vi "set RP100 voltage.vi"(8 "error in (no error)":errorcluster, 10 "字符串 2":string, 11 "config":T1={"initialize"=enum."SR830", "6221"={"6221 Resource"="GPIB0::24::INSTR", "Delta status"=FALSE, "电流|RMS(A)"=0.0}, "SR830+6221"={"source"=0, "Current(A)"=0.0, "阻抗(Ohm)"=0.0, "SR830 1"=FALSE, "SR830 2"=FALSE, "SR830 3"=FALSE, "SR830 4"=FALSE, "VISA 1"="", "VISA 2"="", "VISA 3"="", "VISA 4"="", "Reserve 1"=-1, "Reserve 2"=-1, "Reserve 3"=-1, "Reserve 4"=-1, "Sensitivity 1"=-1, "Sensitivity 2"=-1, "Sensitivity 3"=-1, "Sensitivity 4"=-1, "量程入 1"=0, "量程入 2"=0, "量程入 3"=0, "量程入 4"=0}, "2400"={"2400"=FALSE, "VISA"="GPIB0::9::INSTR", "Output Level (0)"=1e-05, "Compliance  Level (0.1)"=10.0, "ch"=[]}, "ch"={"ch"=[], "current"=[], "change?"=[], "holding current\nwhen change ch?"=FALSE, "current offset"=[]}, "Instrument"={"limit"={"Field limit"=0.0, "Field rate limit"=0.0, "Temp limit"=0.0, "Temp low limit"=0.0, "Temp rate limit "=0.0}, "genarl"={"行数"=refnum, "编辑列表框？"=refnum, "列表框"=refnum, "camg 振荡状态"=refnum, "Aborting"=refnum, "数据文件"=refnum, "warning"=refnum, "vi路径"="", "Instrument Type"=enum."PPMS-Rotate"}, "cmag"={"TM620"="TCPIP0::192.168.1.5::4266::SOCKET", "M24C Resource"="GPIB0::24::INSTR", "4G supply"="", "Temp Status 24C"=refnum, "Temp"=refnum, "9T信号"=refnum, "4g supply status"=refnum, "in-plane"="", "out-plane"="", "in-plane signal"=FALSE, "out-plane signal"=FALSE, "in plane 信号"=refnum, "pzt volt"=refnum, "camg Rate"=refnum}, "lengtou2"={"750 visa"="", "750 rotate"="", "semaphore 340"=refnum, "semaphore 750"=refnum, "750 field status"=refnum, "Input (0:A) 340"=0, "340 Resource"="GPIB0::14::INSTR", "340 Status"=refnum, "Input (0:B) 340"=1, "Loop (0: 1)"=0, "Loop (1: 1)"=0, "TCP master instance"=refnum}, "lengtou"={"TCP master instance"=refnum, "335 Status"=refnum, "335 Resource "="GPIB0::24::INSTR", "Input (0:A) 335"=0, "Input (0:B) 335"=1, "Heater Output (1:1) 335"=1, "semaphore 335"=refnum}, "325 for test"={"quantum design"=refnum, "semaphore 325"=refnum, "325 Resource "="GPIB0::13::INSTR", "Input (0:A) 325"=0, "Heater Output (1:1) 325"=1, "325 Status"=refnum}}, "2614B"={"2614B chA"=FALSE, "2614B chB"=FALSE, "VISA"=""}, "33522b"={"33522b resource name"="GPIB0::16::INSTR", "零电压"=0.0, "最大电压"=148.0, "间隔"=4.0, "最小电压"=-48.0, "loop"=0.0, "压电陶瓷电压(Vpp)"=0.0}, "gating type"=enum."2614(daul)", "层数"=0, "行数"=0, "是否处理"=[], "current 2"=[], "StrainCell"={"RP100 resource name"="GPIB0::16::INSTR", "E4980 resource name"="GPIB0::16::INSTR", "RP100 Reset ?(True)"=TRUE, "Voltage1(V)"=0.0, "Voltage2(V)"=148.0, "interval"=4.0, "slew(V/s)"=-48.0}} {"Instrument"."325 for test"."Heater Output (1:1) 325" items=["1"=1, "2"=2]; "Instrument"."325 for test"."Input (0:A) 325" items=["A", "B"]; "Instrument"."lengtou"."Heater Output (1:1) 335" items=["1"=1, "2"=2]; "Instrument"."lengtou"."Input (0:B) 335" items=["A", "B"]; "Instrument"."lengtou"."Input (0:A) 335" items=["A", "B"]; "Instrument"."lengtou2"."Loop (1: 1)" items=["1", "2"]; "Instrument"."lengtou2"."Loop (0: 1)" items=["1", "2"]; "Instrument"."lengtou2"."Input (0:B) 340" items=["A", "B", "C", "D"]; "Instrument"."lengtou2"."Input (0:A) 340" items=["A", "B", "C", "D"]; "SR830+6221"."Sensitivity 4" items=["Auto Gain"=-1, "2 nV/fA"=0, "5 nV/fA"=1, "10 nV/fA"=2, "20 nV/fA"=3, "50 nV/fA"=4, "100 nV/fA"=5, "200 nV/fA"=6, "500 nV/fA"=7, "1 uV/pA"=8, "2 uV/pA"=9, "5 uV/pA"=10, "10 uV/pA"=11, "20 uV/pA"=12, "50 uV/pA"=13, "100 uV/pA"=14, "200 uV/pA"=15, "500 uV/pA"=16, "1 mV/nA"=17, "2 mV/nA"=18, "5 mV/nA"=19, "10 mV/nA"=20, "20 mV/nA"=21, "50 mV/nA"=22, "100 mV/nA"=23, "200 mV/nA"=24, "500 mV/mA"=25, "1 V/uA"=26]; "SR830+6221"."Sensitivity 3" items=["Auto Gain"=-1, "2 nV/fA"=0, "5 nV/fA"=1, "10 nV/fA"=2, "20 nV/fA"=3, "50 nV/fA"=4, "100 nV/fA"=5, "200 nV/fA"=6, "500 nV/fA"=7, "1 uV/pA"=8, "2 uV/pA"=9, "5 uV/pA"=10, "10 uV/pA"=11, "20 uV/pA"=12, "50 uV/pA"=13, "100 uV/pA"=14, "200 uV/pA"=15, "500 uV/pA"=16, "1 mV/nA"=17, "2 mV/nA"=18, "5 mV/nA"=19, "10 mV/nA"=20, "20 mV/nA"=21, "50 mV/nA"=22, "100 mV/nA"=23, "200 mV/nA"=24, "500 mV/mA"=25, "1 V/uA"=26]; "SR830+6221"."Sensitivity 1" items=["Auto Gain"=-1, "2 nV/fA"=0, "5 nV/fA"=1, "10 nV/fA"=2, "20 nV/fA"=3, "50 nV/fA"=4, "100 nV/fA"=5, "200 nV/fA"=6, "500 nV/fA"=7, "1 uV/pA"=8, "2 uV/pA"=9, "5 uV/pA"=10, "10 uV/pA"=11, "20 uV/pA"=12, "50 uV/pA"=13, "100 uV/pA"=14, "200 uV/pA"=15, "500 uV/pA"=16, "1 mV/nA"=17, "2 mV/nA"=18, "5 mV/nA"=19, "10 mV/nA"=20, "20 mV/nA"=21, "50 mV/nA"=22, "100 mV/nA"=23, "200 mV/nA"=24, "500 mV/mA"=25, "1 V/uA"=26]; "SR830+6221"."Sensitivity 2" items=["Auto Gain"=-1, "2 nV/fA"=0, "5 nV/fA"=1, "10 nV/fA"=2, "20 nV/fA"=3, "50 nV/fA"=4, "100 nV/fA"=5, "200 nV/fA"=6, "500 nV/fA"=7, "1 uV/pA"=8, "2 uV/pA"=9, "5 uV/pA"=10, "10 uV/pA"=11, "20 uV/pA"=12, "50 uV/pA"=13, "100 uV/pA"=14, "200 uV/pA"=15, "500 uV/pA"=16, "1 mV/nA"=17, "2 mV/nA"=18, "5 mV/nA"=19, "10 mV/nA"=20, "20 mV/nA"=21, "50 mV/nA"=22, "100 mV/nA"=23, "200 mV/nA"=24, "500 mV/mA"=25, "1 V/uA"=26]; "SR830+6221"."Reserve 4" items=["Auto Reserve"=-1, "High Reserve"=0, "Normal"=1, "Low Noise"=2]; "SR830+6221"."Reserve 3" items=["Auto Reserve"=-1, "High Reserve"=0, "Normal"=1, "Low Noise"=2]; "SR830+6221"."Reserve 2" items=["Auto Reserve"=-1, "High Reserve"=0, "Normal"=1, "Low Noise"=2]; "SR830+6221"."Reserve 1" items=["Auto Reserve"=-1, "High Reserve"=0, "Normal"=1, "Low Noise"=2]; "SR830+6221"."source" items=["SR830 1", "SR830 2", "SR830 3", "SR830 4"]}) -> (0 "error out":errorcluster, 3 "输出簇":T1={"initialize"=enum."SR830", "6221"={"6221 Resource"="GPIB0::24::INSTR", "Delta status"=FALSE, "电流|RMS(A)"=0.0}, "SR830+6221"={"source"=0, "Current(A)"=0.0, "阻抗(Ohm)"=0.0, "SR830 1"=FALSE, "SR830 2"=FALSE, "SR830 3"=FALSE, "SR830 4"=FALSE, "VISA 1"="", "VISA 2"="", "VISA 3"="", "VISA 4"="", "Reserve 1"=-1, "Reserve 2"=-1, "Reserve 3"=-1, "Reserve 4"=-1, "Sensitivity 1"=-1, "Sensitivity 2"=-1, "Sensitivity 3"=-1, "Sensitivity 4"=-1, "量程入 1"=0, "量程入 2"=0, "量程入 3"=0, "量程入 4"=0}, "2400"={"2400"=FALSE, "VISA"="GPIB0::9::INSTR", "Output Level (0)"=1e-05, "Compliance  Level (0.1)"=10.0, "ch"=[]}, "ch"={"ch"=[], "current"=[], "change?"=[], "holding current\nwhen change ch?"=FALSE, "current offset"=[]}, "Instrument"={"limit"={"Field limit"=0.0, "Field rate limit"=0.0, "Temp limit"=0.0, "Temp low limit"=0.0, "Temp rate limit "=0.0}, "genarl"={"行数"=refnum, "编辑列表框？"=refnum, "列表框"=refnum, "camg 振荡状态"=refnum, "Aborting"=refnum, "数据文件"=refnum, "warning"=refnum, "vi路径"="", "Instrument Type"=enum."PPMS-Rotate"}, "cmag"={"TM620"="GPIB0::24::INSTR", "M24C Resource"="GPIB0::24::INSTR", "4G supply"="GPIB0::24::INSTR", "Temp Status 24C"=refnum, "Temp"=refnum, "9T信号"=refnum, "4g supply status"=refnum, "in-plane"="", "out-plane"="", "in-plane signal"=FALSE, "out-plane signal"=FALSE, "in plane 信号"=refnum, "pzt volt"=refnum, "camg Rate"=refnum}, "lengtou2"={"750 visa"="", "750 rotate"="", "semaphore 340"=refnum, "semaphore 750"=refnum, "750 field status"=refnum, "Input (0:A) 340"=1, "340 Resource"="GPIB0::14::INSTR", "340 Status"=refnum, "Input (0:B) 340"=0, "Loop (0: 1)"=1, "Loop (1: 1)"=0, "TCP master instance"=refnum}, "lengtou"={"TCP master instance"=refnum, "335 Status"=refnum, "335 Resource "="GPIB0::24::INSTR", "Input (0:A) 335"=0, "Input (0:B) 335"=0, "Heater Output (1:1) 335"=0, "semaphore 335"=refnum}, "325 for test"={"quantum design"=refnum, "semaphore 325"=refnum, "325 Resource "="GPIB0::13::INSTR", "Input (0:A) 325"=1000, "Heater Output (1:1) 325"=1, "325 Status"=refnum}}, "2614B"={"2614B chA"=FALSE, "2614B chB"=FALSE, "VISA"=""}, "33522b"={"33522b resource name"="GPIB0::16::INSTR", "零电压"=0.0, "最大电压"=148.0, "间隔"=4.0, "最小电压"=-48.0, "loop"=0.0, "压电陶瓷电压(Vpp)"=0.0}, "gating type"=enum."2614(daul)", "层数"=0, "行数"=0, "是否处理"=[], "current 2"=[], "StrainCell"={"RP100 resource name"="GPIB0::16::INSTR", "E4980 resource name"="GPIB0::16::INSTR", "RP100 Reset ?(True)"=TRUE, "Voltage1(V)"=0.0, "Voltage2(V)"=0.0, "interval"=4.0, "slew(V/s)"=1.0}} {"Instrument"."325 for test"."Heater Output (1:1) 325" items=["1"=1, "2"=2]; "Instrument"."325 for test"."Input (0:A) 325" items=["A", "B"]; "Instrument"."lengtou"."Heater Output (1:1) 335" items=["1"=1, "2"=2]; "Instrument"."lengtou"."Input (0:B) 335" items=["A", "B"]; "Instrument"."lengtou"."Input (0:A) 335" items=["A", "B"]; "Instrument"."lengtou2"."Loop (1: 1)" items=["1", "2"]; "Instrument"."lengtou2"."Loop (0: 1)" items=["1", "2"]; "Instrument"."lengtou2"."Input (0:B) 340" items=["A", "B", "C", "D"]; "Instrument"."lengtou2"."Input (0:A) 340" items=["A", "B", "C", "D"]; "SR830+6221"."Sensitivity 4" items=["Auto Gain"=-1, "2 nV/fA"=0, "5 nV/fA"=1, "10 nV/fA"=2, "20 nV/fA"=3, "50 nV/fA"=4, "100 nV/fA"=5, "200 nV/fA"=6, "500 nV/fA"=7, "1 uV/pA"=8, "2 uV/pA"=9, "5 uV/pA"=10, "10 uV/pA"=11, "20 uV/pA"=12, "50 uV/pA"=13, "100 uV/pA"=14, "200 uV/pA"=15, "500 uV/pA"=16, "1 mV/nA"=17, "2 mV/nA"=18, "5 mV/nA"=19, "10 mV/nA"=20, "20 mV/nA"=21, "50 mV/nA"=22, "100 mV/nA"=23, "200 mV/nA"=24, "500 mV/mA"=25, "1 V/uA"=26]; "SR830+6221"."Sensitivity 3" items=["Auto Gain"=-1, "2 nV/fA"=0, "5 nV/fA"=1, "10 nV/fA"=2, "20 nV/fA"=3, "50 nV/fA"=4, "100 nV/fA"=5, "200 nV/fA"=6, "500 nV/fA"=7, "1 uV/pA"=8, "2 uV/pA"=9, "5 uV/pA"=10, "10 uV/pA"=11, "20 uV/pA"=12, "50 uV/pA"=13, "100 uV/pA"=14, "200 uV/pA"=15, "500 uV/pA"=16, "1 mV/nA"=17, "2 mV/nA"=18, "5 mV/nA"=19, "10 mV/nA"=20, "20 mV/nA"=21, "50 mV/nA"=22, "100 mV/nA"=23, "200 mV/nA"=24, "500 mV/mA"=25, "1 V/uA"=26]; "SR830+6221"."Sensitivity 1" items=["Auto Gain"=-1, "2 nV/fA"=0, "5 nV/fA"=1, "10 nV/fA"=2, "20 nV/fA"=3, "50 nV/fA"=4, "100 nV/fA"=5, "200 nV/fA"=6, "500 nV/fA"=7, "1 uV/pA"=8, "2 uV/pA"=9, "5 uV/pA"=10, "10 uV/pA"=11, "20 uV/pA"=12, "50 uV/pA"=13, "100 uV/pA"=14, "200 uV/pA"=15, "500 uV/pA"=16, "1 mV/nA"=17, "2 mV/nA"=18, "5 mV/nA"=19, "10 mV/nA"=20, "20 mV/nA"=21, "50 mV/nA"=22, "100 mV/nA"=23, "200 mV/nA"=24, "500 mV/mA"=25, "1 V/uA"=26]; "SR830+6221"."Sensitivity 2" items=["Auto Gain"=-1, "2 nV/fA"=0, "5 nV/fA"=1, "10 nV/fA"=2, "20 nV/fA"=3, "50 nV/fA"=4, "100 nV/fA"=5, "200 nV/fA"=6, "500 nV/fA"=7, "1 uV/pA"=8, "2 uV/pA"=9, "5 uV/pA"=10, "10 uV/pA"=11, "20 uV/pA"=12, "50 uV/pA"=13, "100 uV/pA"=14, "200 uV/pA"=15, "500 uV/pA"=16, "1 mV/nA"=17, "2 mV/nA"=18, "5 mV/nA"=19, "10 mV/nA"=20, "20 mV/nA"=21, "50 mV/nA"=22, "100 mV/nA"=23, "200 mV/nA"=24, "500 mV/mA"=25, "1 V/uA"=26]; "SR830+6221"."Reserve 4" items=["Auto Reserve"=-1, "High Reserve"=0, "Normal"=1, "Low Noise"=2]; "SR830+6221"."Reserve 3" items=["Auto Reserve"=-1, "High Reserve"=0, "Normal"=1, "Low Noise"=2]; "SR830+6221"."Reserve 2" items=["Auto Reserve"=-1, "High Reserve"=0, "Normal"=1, "Low Noise"=2]; "SR830+6221"."Reserve 1" items=["Auto Reserve"=-1, "High Reserve"=0, "Normal"=1, "Low Noise"=2]; "SR830+6221"."source" items=["SR830 1", "SR830 2", "SR830 3", "SR830 4"]})   [LabVIEW 2019, in "nematic.lvlib" / "Copy of StrainCell.lvlib"]
uses:
  nematic/Copy of StrainCell.lvlib
  ctl/config.ctl
  <vilib>/NI/Modbus Library/API/Master/Modbus Master.lvclass
  ctl/initialize.ctl
  ctl/Instrument.ctl
  ctl/limit.ctl
  ctl/warning.ctl
  ctl/Instrument Type.ctl
  ctl/335 state.ctl
  ctl/9T mag field stauts.ctl
  C:/Users/fuyang/Desktop/postdoctor/labview/labview-measure/lib/QDInstrument.dll
  lib/QDInstrument.dll
  ctl/Gating type.ctl
  lib/RP100/RP100.lvlib
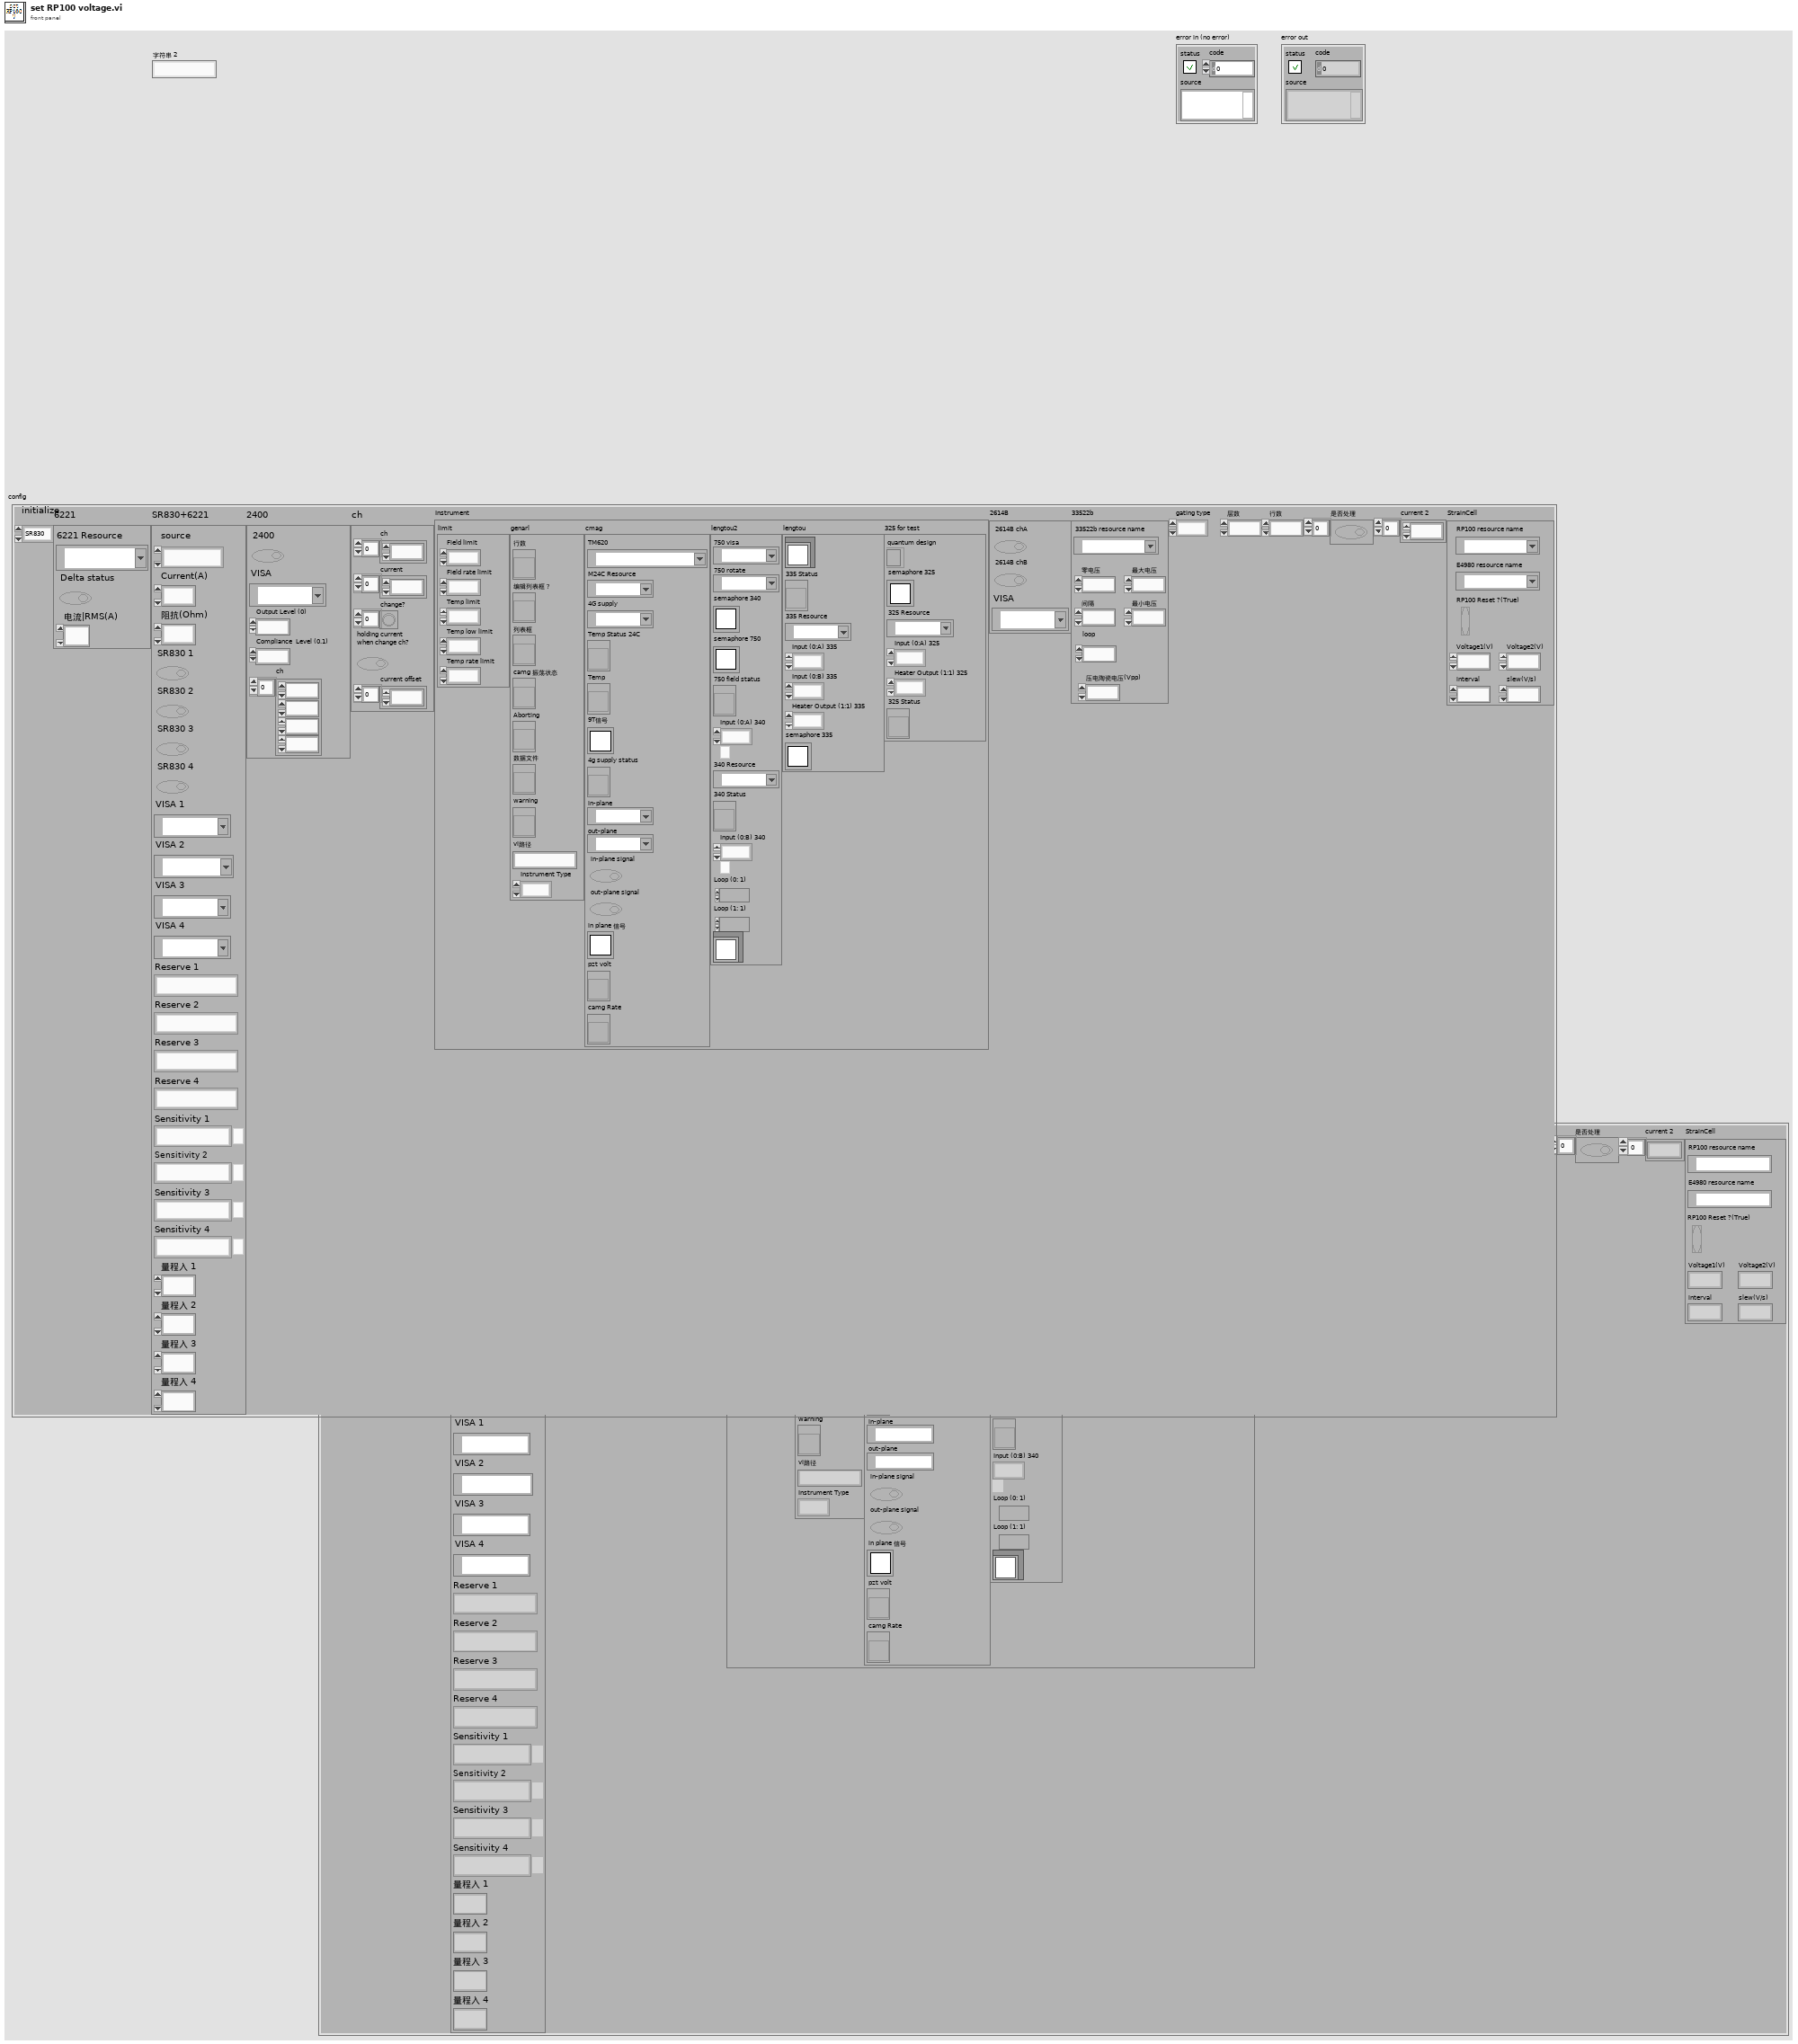
[diagram p1: front panel]
types:
  T1 = typedef "config.ctl" = cluster{"initialize":T2, "6221":cluster{"6221 Resource":refnum<visa-resource-name>, "Delta status":bool, "电流|RMS(A)":dbl}, "SR830+6221":cluster{"source":u16, "Current(A)":dbl, "阻抗(Ohm)":dbl, "SR830 1":bool, "SR830 2":bool, "SR830 3":bool, "SR830 4":bool, "VISA 1":refnum<visa-resource-name>, "VISA 2":refnum<visa-resource-name>, "VISA 3":refnum<visa-resource-name>, "VISA 4":refnum<visa-resource-name>, "Reserve 1":i16, "Reserve 2":i16, "Reserve 3":i16, "Reserve 4":i16, "Sensitivity 1":i16, "Sensitivity 2":i16, "Sensitivity 3":i16, "Sensitivity 4":i16, "量程入 1":i32, "量程入 2":i32, "量程入 3":i32, "量程入 4":i32}, "2400":cluster{"2400":bool, "VISA":refnum<visa-resource-name>, "Output Level (0)":dbl, "Compliance  Level (0.1)":dbl, "ch":i32[]}, "ch":cluster{"ch":i32[], "current":dbl[], "change?":bool[], "holding current\nwhen change ch?":bool, "current offset":dbl[]}, "Instrument":T3, "2614B":cluster{"2614B chA":bool, "2614B chB":bool, "VISA":refnum<visa-resource-name>}, "33522b":cluster{"33522b resource name":refnum<visa-resource-name>, "零电压":dbl, "最大电压":dbl, "间隔":dbl, "最小电压":dbl, "loop":dbl, "压电陶瓷电压(Vpp)":dbl}, "gating type":T7, "层数":i32, "行数":i32, "是否处理":bool[], "current 2":dbl[], "StrainCell":cluster{"RP100 resource name":refnum<visa-resource-name>, "E4980 resource name":refnum<visa-resource-name>, "RP100 Reset ?(True)":bool, "Voltage1(V)":dbl, "Voltage2(V)":dbl, "interval":dbl, "slew(V/s)":dbl}}
  T2 = typedef "initialize.ctl" = enum16{"SR830", "keithley6221-SR830", "Delta", "Delta-tunnelling", "keithley6221-2182-DC", "PZT", "StrainCell", "4200"}
  T3 = typedef "Instrument.ctl" = cluster{"limit":T4, "genarl":cluster{"行数":refnum<vi>, "编辑列表框？":refnum<vi>, "列表框":refnum<vi>, "camg 振荡状态":refnum<vi>, "Aborting":refnum<vi>, "数据文件":refnum<vi>, "warning":refnum<vi>, "vi路径":string, "Instrument Type":T5}, "cmag":cluster{"TM620":refnum<visa-resource-name>, "M24C Resource":refnum<visa-resource-name>, "4G supply":refnum<visa-resource-name>, "Temp Status 24C":refnum<vi>, "Temp":refnum<vi>, "9T信号":T6, "4g supply status":refnum<vi>, "in-plane":refnum<visa-resource-name>, "out-plane":refnum<visa-resource-name>, "in-plane signal":bool, "out-plane signal":bool, "in plane 信号":T6, "pzt volt":refnum<vi>, "camg Rate":refnum<vi>}, "lengtou2":cluster{"750 visa":refnum<visa-resource-name>, "750 rotate":refnum<visa-resource-name>, "semaphore 340":T6, "semaphore 750":T6, "750 field status":refnum<vi>, "Input (0:A) 340":u16, "340 Resource":refnum<visa-resource-name>, "340 Status":refnum<vi>, "Input (0:B) 340":u16, "Loop (0: 1)":u16, "Loop (1: 1)":u16, "TCP master instance":refnum<class "Modbus Master.lvclass">}, "lengtou":cluster{"TCP master instance":refnum<class "Modbus Master.lvclass">, "335 Status":refnum<vi>, "335 Resource ":refnum<visa-resource-name>, "Input (0:A) 335":u16, "Input (0:B) 335":u16, "Heater Output (1:1) 335":u16, "semaphore 335":T6}, "325 for test":cluster{"quantum design":refnum<k24>, "semaphore 325":T6, "325 Resource ":refnum<visa-resource-name>, "Input (0:A) 325":u16, "Heater Output (1:1) 325":u16, "325 Status":refnum<vi>}}
  T4 = typedef "limit.ctl" = cluster{"Field limit":dbl, "Field rate limit":dbl, "Temp limit":dbl, "Temp low limit":dbl, "Temp rate limit ":dbl}
  T5 = typedef "Instrument Type.ctl" = enum16{"PPMS", "VersaLab", "DynaCool", "SVSM", "PPMS-Rotate", "Lakeshore335", "lengtou2", "9T mag old", "9T cmag", "9T cmag DAC", "9T cmag rotate", "test"}
  T6 = typedef "Semaphore RefNum" = refnum<k1>
  T7 = typedef "Gating type.ctl" = enum32{"null", "2614(daul)", "2400", "6517B"}
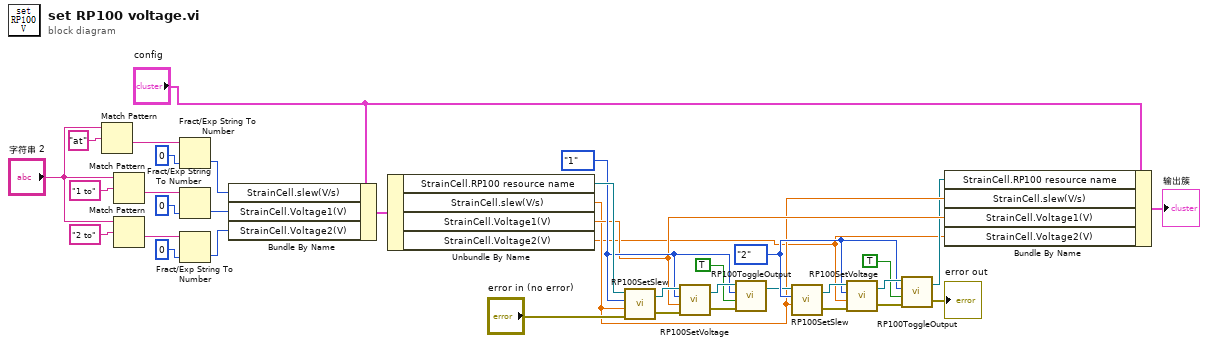
[diagram p0: block diagram]
diagram:
  w12 = enum16{"1", "2", "Both"}."2" ("Source")
  w19 = enum16{"1", "2", "Both"}."1" ("Source")
  n1 = Match Pattern(string="字符串 2", regular expression="at" ("正则表达式")) -> (after substring=w27:string)  [unwired: 1 in, 3 out]
  n2 = Match Pattern(string="字符串 2", regular expression="1 to" ("正则表达式")) -> (after substring=w30:string)  [unwired: 1 in, 3 out]
  n3 = Match Pattern(string="字符串 2", regular expression="2 to" ("正则表达式")) -> (after substring=w9:string)  [unwired: 1 in, 3 out]
  n4 = Fract/Exp String To Number(string=w27, default (0 dbl)=0) -> (number=w26:i32)  [unwired: 2 in, 1 out]
  n5 = Fract/Exp String To Number(string=w30, default (0 dbl)=0) -> (number=w25:i32)  [unwired: 2 in, 1 out]
  n6 = Fract/Exp String To Number(string=w9, default (0 dbl)=0) -> (number=w6:i32)  [unwired: 2 in, 1 out]
  n7 = Bundle By Name(cluster="config", "StrainCell.slew(V/s)"=w26, "StrainCell.Voltage1(V)"=w25, "StrainCell.Voltage2(V)"=w6) -> (w24:T1)
  n8 = Unbundle By Name(w24) -> ("StrainCell.RP100 resource name"=w33:refnum<visa-resource-name>, "StrainCell.slew(V/s)"=w5:dbl, "StrainCell.Voltage1(V)"=w18:dbl, "StrainCell.Voltage2(V)"=w2:dbl)
  n9 = call "RP100SetSlew.vi"("error in (no error)"="error in (no error)", "Slew"=w5, "Source"=w19, "VISA resource name"=w33) -> ("error out"=w35:errorcluster, "VISA resource name out"=w36:refnum<visa-resource-name>)
  n10 = call "RP100SetVoltage.vi"("error in (no error)"=w35, "Voltage"=w18, "Source"=w19, "VISA resource name"=w36) -> ("error out"=w20:errorcluster, "VISA resource name out"=w22:refnum<visa-resource-name>)
  n11 = call "RP100ToggleOutput.vi"("error in (no error)"=w20, "Enable?"=TRUE, "Source"=w19, "VISA resource name"=w22) -> ("VISA resource name out"=w11:refnum<visa-resource-name>)  [unwired: 1 out]
  n12 = call "RP100SetSlew.vi"("Slew"=w5, "Source"=w12, "VISA resource name"=w11) -> ("error out"=w16:errorcluster, "VISA resource name out"=w17:refnum<visa-resource-name>)  [unwired: 1 in]
  n13 = call "RP100SetVoltage.vi"("error in (no error)"=w16, "Voltage"=w2, "Source"=w12, "VISA resource name"=w17) -> ("error out"=w13:errorcluster, "VISA resource name out"=w15:refnum<visa-resource-name>)
  n14 = call "RP100ToggleOutput.vi"("error in (no error)"=w13, "Enable?"=TRUE, "Source"=w12, "VISA resource name"=w15) -> ("error out"=→"error out":errorcluster, "VISA resource name out"=w3:refnum<visa-resource-name>)
  n15 = Bundle By Name(cluster="config", "StrainCell.RP100 resource name"=w3, "StrainCell.slew(V/s)"=w5, "StrainCell.Voltage1(V)"=w18, "StrainCell.Voltage2(V)"=w2) -> (→"输出簇":T1)
